vi "Main.vi"() -> ()   [LabVIEW 2013]
uses:
  <vilib>/Utility/error.llb/DialogType.ctl
panel:
  out "Conn status":bool caption="NC"
  in  "Выкл.":bool
  in  "IP":string="172.16.21.120"
  out "conn src":refnum<k5>
  in  "stop":bool
  out "message":string=" INSTRUCTIONS:\r\rNormal Use:  When using subVIs that incorporate the error in/error out (or error I/O) structure, place this handler where you want to inform the user of an error, typically at the end of the I/O data path, as the last action of the program.  If the error in error? is ERROR, the handler creates a message describing the error and its source.  If the type of dialog = 1 (default), the message is displayed to the user, who can only acknowedge it.  If the type = 2, the user can acknowledge the message or abort execution; aborting a program with active I/O is not recommended.  If the type = 0, no message is displayed; this is used to process the error programmatically, and the error out cluster elements are wired to individual terminals for that reason.  \r\rOther Use:\n\r\nlocal testing.  To test the error code of a subVI or function that does not have the error I/O structure, you can wire its error code and a source string to the local error code and error source inputs.  If error in error? indicates no error and error code is not equal to 0, the local code and source are substituted for the error in values, and error? is set TRUE (ERROR)."
  in  "V":dbl min=0.0 max=30.0 step=1.0 format="%.1f"
  in  "А":dbl min=0.0 max=300.0 step=0.001 format="%.3f"
  in  "NeedToSetVoltage":bool
  in  "NeedToSetCurrent":bool
  out "V":string
  out "А":string
  in  "вкл.":bool
  out "Out":bool
  # "HILAC beam bending magnet supply"
  # "Settings"
  # "Voltage"
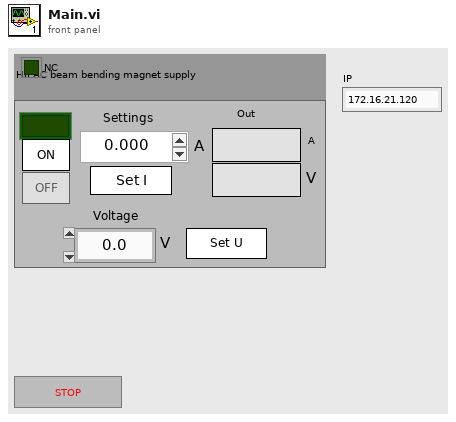
[diagram p1: front panel]
types:
  T1 = enum8{"Enabled", "Disabled", "Disabled and Grayed Out"}
  T2 = typedef "DialogType.ctl" = u16
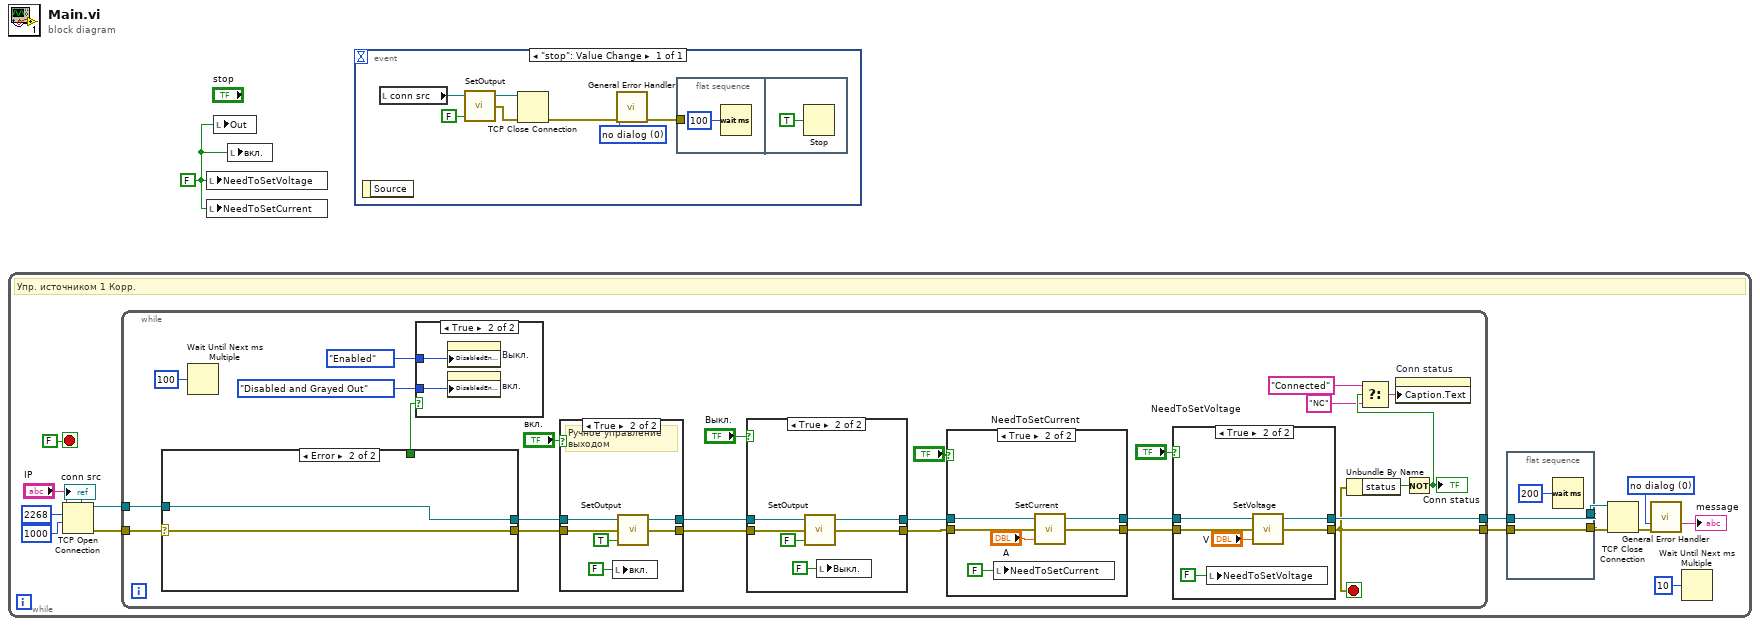
[diagram p0: block diagram]
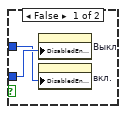
[diagram p2: hidden frame]
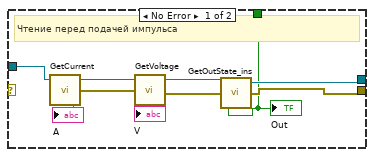
[diagram p6: hidden frame]
diagram:
  w1 = FALSE ("Connect")
  n1 = while {
    stop <- FALSE stop-if-true
    w10 = T2 0 items=["no dialog", "OK message", "continue or stop message", "OK message + warnings", "continue/stop + warnings"] ("type of dialog (OK msg:1)")
    # "Упр. источником 1 Корр."
    n2 = TCP Open Connection(address="IP", remote port or service name=u16 2268 ("Port"), timeout ms (60000)=1000) -> (connection ID=w12:refnum<k5>, error out=w13:errorcluster)  [unwired: 1 in, 1 out]
    "conn src" <- w12
    n3 = while {
      tunnel: w13 -> [w43]
      tunnel: w12 -> [w42]
      tunnel: [w41] -> w5
      tunnel: [w27] -> w4
      stop <- w27 stop-if-true
      n4 = case shown="Error" w43 {
        selector: w43 -> [_ w82]
        tunnel: w42 -> [w77 w83]
        tunnel: [w73 w82] -> w37
        tunnel: [w74 w83] -> w36
        tunnel: [w72 _] -> w19
        frame No Error {
          # "Чтение перед подачей импульса"
          n5 = call "GetCurrent.vi"("connection ID"=w77) -> ("Current"=→"А":string, "error out"=w78:errorcluster, "connection ID out"=w80:refnum<k5>)  [unwired: 1 in, 1 out]
          n6 = call "GetVoltage.vi"("error in"=w78, "connection ID"=w80) -> ("Voltage"=→"V":string, "error out"=w75:errorcluster, "connection ID out"=w76:refnum<k5>)  [unwired: 1 out]
          n7 = call "GetOutState_ins.vi"("error in"=w75, "connection ID"=w76) -> ("error out"=w73:errorcluster, "connection ID out"=w74:refnum<k5>, "Answer"=w72:bool)  [unwired: 1 in]
          "Out" <- w72
        }
        frame Error {
        }
      }
      n8 = Wait Until Next ms Multiple(millisecond multiple=u32 100) -> ()  [unwired: 1 out]
      n9 = case shown="True" w19 {
        tunnel: T1."Enabled" ("Disabled") -> [w44 w47]
        tunnel: T1."Disabled and Grayed Out" ("Disabled") -> [w45 w46]
        frame False {
          n10 = property on="Выкл." class="Bool (strict)"("DisabledEnum"=w45) -> ()  [unwired: 2 in, 2 out]
          n11 = property on="вкл." class="Bool (strict)"("DisabledEnum"=w44) -> ()  [unwired: 2 in, 2 out]
        }
        frame True {
          n12 = property on="Выкл." class="Bool (strict)"("DisabledEnum"=w47) -> ()  [unwired: 2 in, 2 out]
          n13 = property on="вкл." class="Bool (strict)"("DisabledEnum"=w46) -> ()  [unwired: 2 in, 2 out]
        }
      }
      n14 = case shown="True" "вкл." {
        tunnel: w37 -> [w64 w71]
        tunnel: w36 -> [w65 w70]
        tunnel: [w65 w68] -> w31
        tunnel: [w64 w67] -> w30
        frame False {
        }
        frame True {
          # "Ручное управление выходом"
          n15 = local write "вкл."(FALSE ("вкл.")) -> ()
          n16 = call "SetOutput.vi"("State"=TRUE, "error in"=w71, "connection ID"=w70) -> ("error out"=w67:errorcluster, "connection ID out"=w68:refnum<k5>)  [unwired: 1 out]
        }
      }
      n17 = case shown="True" "Выкл." {
        tunnel: w31 -> [w49 w54]
        tunnel: w30 -> [w48 w53]
        tunnel: [w49 w51] -> w29
        tunnel: [w48 w50] -> w28
        frame False {
        }
        frame True {
          n18 = call "SetOutput.vi"("State"=FALSE, "error in"=w53, "connection ID"=w54) -> ("error out"=w50:errorcluster, "connection ID out"=w51:refnum<k5>)  [unwired: 1 out]
          n19 = local write "Выкл."(FALSE ("Выкл.")) -> ()
        }
      }
      n20 = case shown="True" "NeedToSetCurrent" {
        tunnel: [w57 w62] -> w40
        tunnel: [w56 w60] -> w38
        tunnel: w29 -> [w57 w59]
        tunnel: w28 -> [w56 w58]
        frame False {
        }
        frame True {
          n21 = local write "NeedToSetCurrent"(FALSE ("NeedToSetOutput")) -> ()
          n22 = call "SetCurrent.vi"("Current"="А", "error in"=w58, "connection ID"=w59) -> ("error out"=w60:errorcluster, "connection ID out"=w62:refnum<k5>)  [unwired: 1 out]
        }
      }
      n23 = case shown="True" "NeedToSetVoltage" {
        tunnel: w40 -> [w85 w91]
        tunnel: [w85 w88] -> w41
        tunnel: w38 -> [w84 w87]
        tunnel: [w84 w86] -> w27
        frame False {
        }
        frame True {
          n24 = local write "NeedToSetVoltage"(FALSE ("NeedToSetOutput")) -> ()
          n25 = call "SetVoltage.vi"("Voltage"="V", "error in"=w87, "connection ID"=w91) -> ("error out"=w86:errorcluster, "connection ID out"=w88:refnum<k5>)  [unwired: 1 out]
        }
      }
      n26 = Unbundle By Name(w27) -> ("status"=w26:bool)
      n27 = Not(x=w26) -> (.not. x?=w23:bool)
      "Conn status" <- w23
      n28 = Select(t="Connected", s=w23, f="NC") -> (s? t:f=w21:string)
      n29 = property on="Conn status" class="Bool (strict)"("Caption.Text"=w21) -> ()  [unwired: 2 in, 2 out]
    }
    n30 = flat-sequence {
      tunnel: [w18] -> w6
      tunnel: w5 -> [w18]
      tunnel: [w17] -> w3
      tunnel: w4 -> [w17]
      frame #0 {
        n31 = Wait (ms)(milliseconds to wait=u32 200 ("millisecond multiple")) -> ()  [unwired: 1 out]
      }
    }
    n32 = TCP Close Connection(connection ID=w6, error in (no error)=w3) -> (error out=w11:errorcluster)  [unwired: 2 out]
    n33 = call <vilib>:"General Error Handler.vi"("type of dialog (OK msg:1)"=w10, "error in (no error)"=w11) -> ("message"=→"message":string)  [unwired: 9 in, 4 out]
    n34 = Wait Until Next ms Multiple(millisecond multiple=u32 10) -> ()  [unwired: 1 out]
  }
  n35 = local write "NeedToSetVoltage"(w1) -> ()
  n36 = local write "NeedToSetCurrent"(w1) -> ()
  n37 = local write "Out"(w1) -> ()
  n38 = local write "вкл."(w1) -> ()
  n39 = event shown="[0] \"stop\": Value Change" {
    selector: _ -> [_]
    dyn-events: _ -> [_]
    timeout: _ -> [_]
    event "stop": Value Change {
      w98 = T2 0 items=["no dialog", "OK message", "continue or stop message", "OK message + warnings", "continue/stop + warnings"] ("type of dialog (OK msg:1)")
      n40 = event-data() -> ()  [unwired: 1 in, 1 out]
      n41 = local read "conn src"() -> (w96:refnum<k5>)
      n42 = call "SetOutput.vi"("State"=FALSE, "connection ID"=w96) -> ("error out"=w94:errorcluster, "connection ID out"=w95:refnum<k5>)  [unwired: 1 in, 1 out]
      n43 = TCP Close Connection(connection ID=w95, error in (no error)=w94) -> (error out=w92:errorcluster)  [unwired: 1 in, 1 out]
      n44 = call <vilib>:"General Error Handler.vi"("type of dialog (OK msg:1)"=w98, "error in (no error)"=w92) -> ("error out"=w97:errorcluster)  [unwired: 9 in, 4 out]
      n45 = flat-sequence {
        tunnel: w97 -> [_]
        frame #0 {
          n46 = Wait (ms)(milliseconds to wait=u32 100) -> ()  [unwired: 1 out]
        }
        frame #1 {
          n47 = Stop(stop? (T)=TRUE) -> ()
        }
      }
    }
  }
